vi "uService GUI.vi"(8 "error in (no error)":errorcluster, 11 "uService Template in":refnum<class "Test_uService.lvclass">) -> (3 "uService Template out":refnum<class "Test_uService.lvclass">)   [LabVIEW 2020, in "Test_uService.lvlib" / "Test_uService.lvclass"]
uses:
  Test_uService.lvclass
  Test_uService.lvclass/Test_uService.ctl
  TALOS/TALOS_PPL.lvlibp/Father of all uServices/Father of all uServices/Father of all uServices.lvclass
  C:/LabVIEW Code/aegis-labview-code/TALOS/TALOS_PPL.lvlibp/Father of all uServices/Father of all uServices/Father of all uServices.lvclass
panel:
  in  "File":bool
  in  "Send to DAQ":bool
  out "Sigma (s)":dbl
  out "Mean trip time (s)":dbl
  out "Echo done":bool
  in  "Target uService":string
  out "Echos performed":u16
  in  "Echos to be performed":u16
  in  "Start echo":bool
  in  "Reset":bool
  in  "Add point":bool
  in  "Tab Control":enum32{"Page 1", "Page 2"}(tab)
  out "Waveform Chart":waveform(dbl)(graph)
  out "Waveform Chart 2":waveform(dbl)(graph)
  in  "stop New uService":bool
  # "I'm the new uService!"
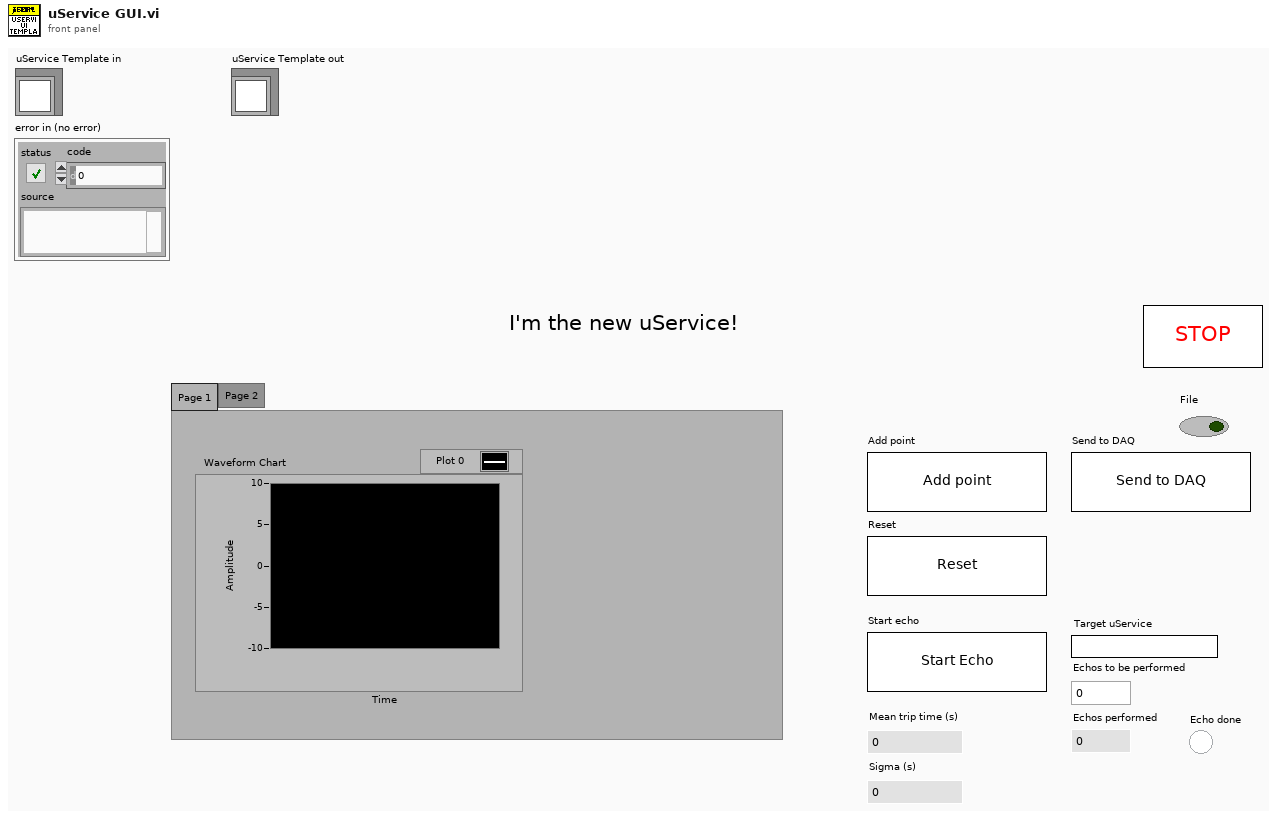
[diagram p1: front panel]
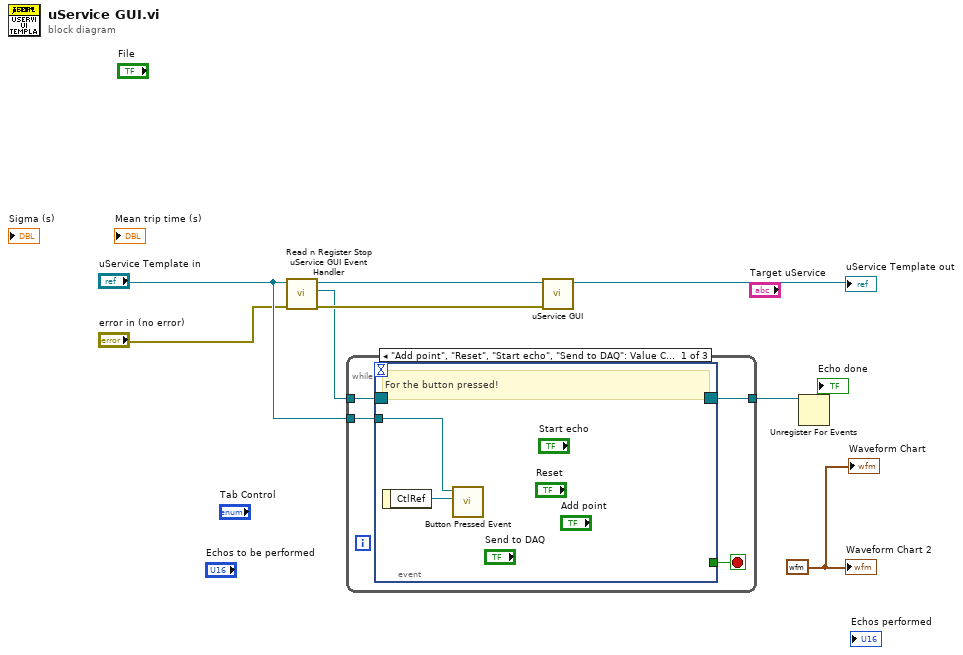
[diagram p0: block diagram]
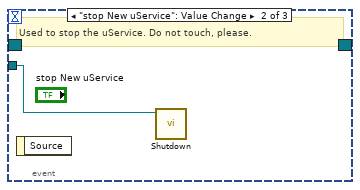
[diagram p2: hidden frame]
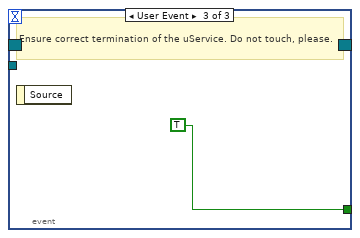
[diagram p3: hidden frame]
diagram:
  w1 = waveform(dbl) {"t0"=timestamp(0 s since 1904-01-01), "dt"=1.0, "Y"=[]} ("Waveform")
  n1 = call-dynamic "Read n Register Stop uService GUI Event Handler .vi"("error in (no error)"="error in (no error)", "uService Template in"="uService Template in") -> ("error out"=w6:errorcluster, "Stop uService GUI Event Ref"=w5:refnum<event-registration>, "uService Template out"=w7:refnum<class "Test_uService.lvclass">)  [unwired: 7 in]
  n2 = while {
    tunnel: [w12] -> w8
    tunnel: w5 -> [w10]
    tunnel: "uService Template in" -> [w9]
    stop <- w11 stop-if-true
    n3 = event shown="[0] \"Add point\", \"Reset\", \"Start echo\", \"Send to DAQ\": Value Change" {
      selector: w10 -> [_ _ _]
      dyn-events: [_ _ _] -> w12
      timeout: _ -> [_ _ _]
      tunnel: [_ _ TRUE] -> w11
      tunnel: w9 -> [w14 w15 _]
      event "Add point", "Reset", "Start echo", "Send to DAQ": Value Change {
        # "For the button pressed!"
        n4 = event-data() -> ("CtlRef"=w13:refnum<vi>)  [unwired: 1 in]
        n5 = call-dynamic "Button Pressed Event.vi"("CtlRef"=w13, "uService Template in"=w14) -> ()  [unwired: 8 in, 2 out]
      }
      event "stop New uService": Value Change {
        # "Used to stop the uService. Do not touch, please."
        n6 = event-data() -> ()  [unwired: 1 in, 1 out]
        n7 = call "Shutdown.vi"("Father of all uServices in"=w15) -> ()  [unwired: 9 in, 2 out]
      }
      event User Event {
        # "Ensure correct termination of the uService. Do not touch, please."
        n8 = event-data() -> ()  [unwired: 1 in, 1 out]
      }
    }
  }
  n9 = call-parent "uService GUI.vi"("error in (no error)"=w6, "uService Template in"=w7) -> ("uService Template out"=→"uService Template out":refnum<class "Test_uService.lvclass">)  [unwired: 9 in]
  n10 = Unregister For Events(event registration refnum=w8) -> ()  [unwired: 1 in, 1 out]
  "Waveform Chart" <- w1
  "Waveform Chart 2" <- w1
